vi "Global.vi"() -> ()   [LabVIEW 2017, in "nifxpmath_NaturalLogarithm.xnode"]
uses:
  <vilib>/rvi/FXPMathLib/FxpLn/XNode/nifxpmath_NaturalLogarithm.xnode
panel:
  in  "TERM UNDEFINED NAME":string="undefined"
  in  "TERM UNDEFINED ID":string="TERM_U"
  out "SMALL ICON w/ 4WIRE":picture
  out "SMALL ICON":picture
  out "NORMAL BANNER":picture
  in  "TERM L NAME":string="ln(x)"
  in  "TERM X NAME":string="x"
  in  "TERM L ID":string="TERM_L"
  in  "TERM X ID":string="TERM_X"
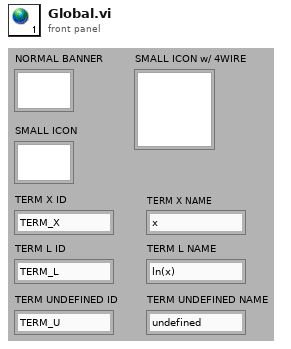
[diagram p1: front panel]
diagram:
